vi "Labspec2Matlab.vi"() -> ()   [LabVIEW 2014]
uses:
  Hardware Control/Spectrometer/Spectrometer Function.ctl
  Save Data/SaveData Function.ctl
  Save Data/SaveData Workspace Info.ctl
  <vilib>/regexp/Match Regular Expression.xnode
panel:
  in  "Convert":bool
  in  "Labspec File":path
  # "LICENSED MATERIALS – PROPERTY OF IBM\nCopyright IBM Corp. 2016,\nALL RIGHTS RESERVED"
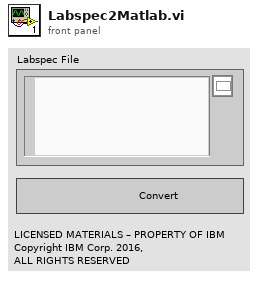
[diagram p1: front panel]
types:
  T1 = typedef "SaveData Function.ctl" = enum16{"Start Python Session", "Set Data Structures to Default", "Append Stress Data", "Append Electrical Measurement", "Append Optical Spectrum", "Append Stress Measurement Step", "Append Instrument Sequence Step", "Set Instrument Configuration", "Set Stress Data", "Set Electrical Measurement", "Set Optical Spectum", "Save Electrical Measurement", "Save Optical Spectrum", "Save Optoelectronic Measurement", "Save Instrument Sequence", "Save Stress Measurement", "Pickle2Workspace", "Explore Variable Space", "Close"}
  T2 = typedef "Spectrometer Function.ctl" = enum16{"Connect", "Complete Configuration", "Get Status", "Load Configuration", "Save Configuration", "Acquire Spectrum", "Read File", "Set Laser", "Set Filter", "Set Hole", "Set Grating", "Set Grating Position", "Set Detector", "Set Acquisition Mode", "Update Refnums", "Disconnect"}
  T3 = typedef "SaveData Workspace Info.ctl" = cluster{"Device Name":string, "Device Info":string, "Path":path}
  T4 = typedef "Spectral Data.ctl" = cluster{"Intensity":dbl[], "Wavelength":dbl[], "Energy":dbl[], "Raman Shift":dbl[], "Detector Temperature":dbl}
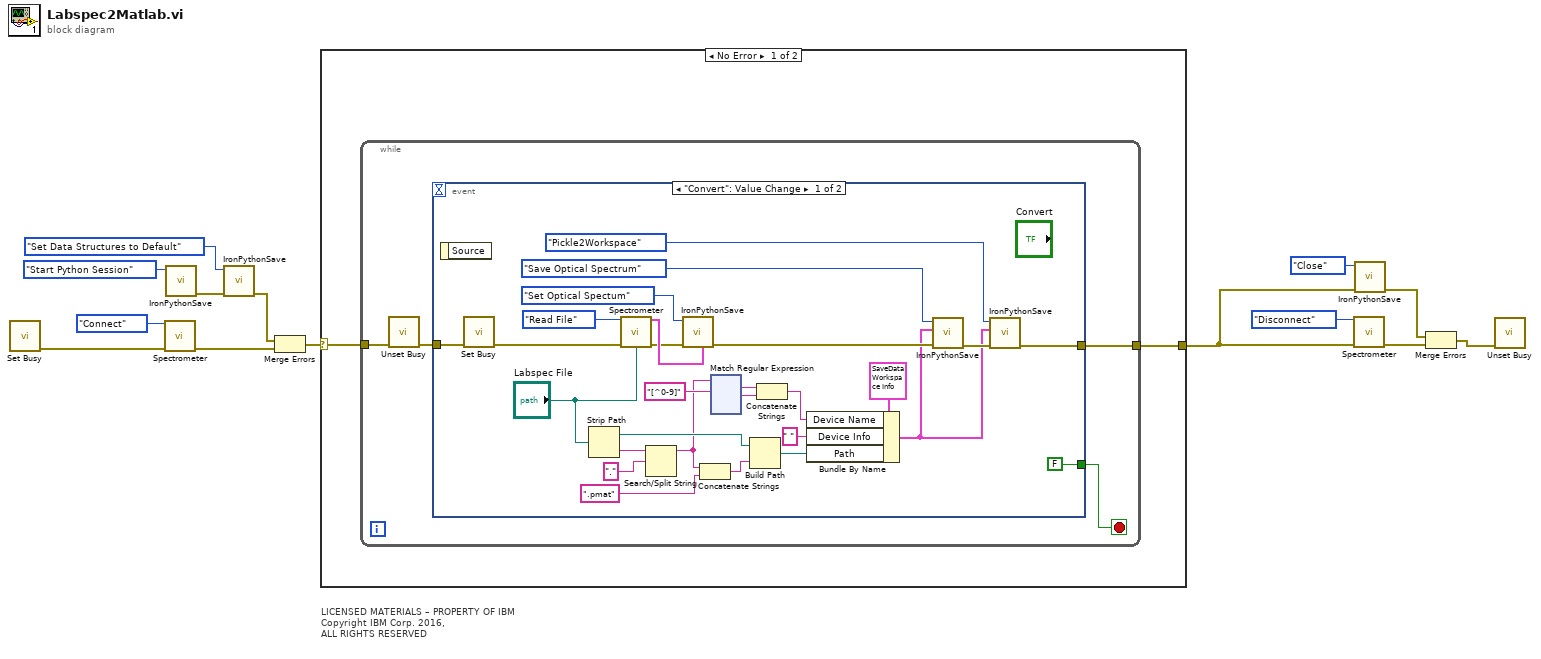
[diagram p0: block diagram]
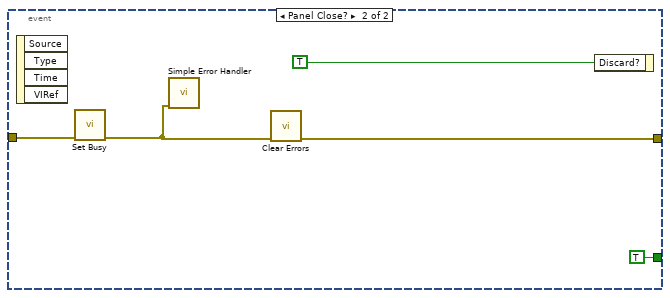
[diagram p2: hidden frame]
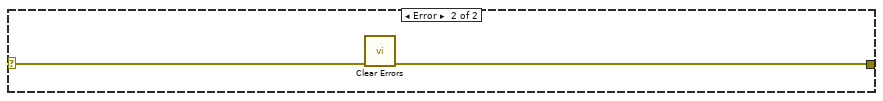
[diagram p3: hidden frame]
diagram:
  # "LICENSED MATERIALS – PROPERTY OF IBM\nCopyright IBM Corp. 2016,\nALL RIGHTS RESERVED"
  n1 = call <vilib>:"Set Busy.vi"() -> ("error out"=w4:errorcluster)  [unwired: 10 in, 1 out]
  n2 = call "Spectrometer.vi"("Function"=Spectrometer_Function."Connect", "error in"=w4) -> ("error out"=w13:errorcluster)  [unwired: 9 in, 4 out]
  n3 = call "IronPythonSave.vi"("Function"=SaveData_Function."Start Python Session") -> ("error out"=w6:errorcluster)  [unwired: 10 in]
  n4 = call "IronPythonSave.vi"("error in (no error)"=w6, "Function"=SaveData_Function."Set Data Structures to Default") -> ("error out"=w5:errorcluster)  [unwired: 9 in]
  n5 = Merge Errors(w5, w13) -> (w11:errorcluster)
  n6 = case shown="No Error" w11 {
    selector: w11 -> [w16 w168]
    tunnel: [w15 w167] -> w8
    frame No Error {
      n7 = while {
        tunnel: w16 -> [w18]
        tunnel: [w20] -> w15
        stop <- w19 stop-if-true
        n8 = call <vilib>:"Unset Busy.vi"("error in (no error)"=w18) -> ("error out"=w17:errorcluster)  [unwired: 10 in]
        n9 = event shown="[0] \"Convert\": Value Change" {
          selector: _ -> [_ _]
          dyn-events: _ -> [_ _]
          timeout: _ -> [_ _]
          tunnel: w17 -> [w27 w165]
          tunnel: [w38 w164] -> w20
          tunnel: [FALSE TRUE] -> w19
          event "Convert": Value Change {
            n10 = event-data() -> ()  [unwired: 1 in, 1 out]
            n11 = call <vilib>:"Set Busy.vi"("error in (no error)"=w27) -> ("error out"=w26:errorcluster)  [unwired: 9 in, 1 out]
            n12 = Strip Path(path="Labspec File") -> (stripped path=w35:path, name=w33:string)
            n13 = call "Spectrometer.vi"("Function"=Spectrometer_Function."Read File", "error in"=w26, "Path"="Labspec File") -> ("Spectrum"=w44:T4, "error out"=w41:errorcluster)  [unwired: 8 in, 3 out]
            n14 = Search/Split String(string=w33, search string/char (-)=".") -> (substring before match=w21:string)  [unwired: 3 out]
            n15 = call "IronPythonSave.vi"("Optical Spectrum"=w44, "error in (no error)"=w41, "Function"=SaveData_Function."Set Optical Spectum") -> ("error out"=w40:errorcluster)  [unwired: 8 in]
            n16 = Concatenate Strings(w21, ".pmat" ("search string/char (-)")) -> (w30:string)
            n17 = xnode "Match Regular Expression"("input string"=w21, "regular expression"="[^0-9]") -> ("whole match"=w24:string, "after match"=w25:string)  [unwired: 4 in, 3 out]
            n18 = Build Path(base path=w35, name or relative path=w30) -> (appended path=w28:path)
            n19 = Concatenate Strings(w24, w25) -> (w23:string)
            n20 = Bundle By Name(cluster=T3 {"Device Name"="test", "Device Info"="test", "Path"=path "C:/Users/gio/Desktop/test Python2Workspace/python2workspace_test.pmat"} ("Workspace Info"), "Device Name"=w23, "Device Info"=" ", "Path"=w28) -> (w32:T3)
            n21 = call "IronPythonSave.vi"("error in (no error)"=w40, "Workspace Info"=w32, "Function"=SaveData_Function."Save Optical Spectrum") -> ("error out"=w39:errorcluster)  [unwired: 8 in]
            n22 = call "IronPythonSave.vi"("error in (no error)"=w39, "Workspace Info"=w32, "Function"=SaveData_Function."Pickle2Workspace") -> ("error out"=w38:errorcluster)  [unwired: 8 in]
          }
          event Panel Close? {
            n23 = event-data() -> ()  [unwired: 1 in, 4 out]
            n24 = call <vilib>:"Set Busy.vi"("error in (no error)"=w165) -> ("error out"=w162:errorcluster)  [unwired: 9 in, 1 out]
            n25 = call <vilib>:"Simple Error Handler.vi"("error in (no error)"=w162) -> ()  [unwired: 4 in, 5 out]
            n26 = call <vilib>:"Clear Errors.vi"("error in (no error)"=w162) -> ("error out"=w164:errorcluster)  [unwired: 5 in, 1 out]
            n27 = event-data("Discard?"=TRUE) -> ()  [unwired: 1 in, 1 out]
          }
        }
      }
    }
    frame Error {
      n28 = call <vilib>:"Clear Errors.vi"("error in (no error)"=w168) -> ("error out"=w167:errorcluster)  [unwired: 5 in, 1 out]
    }
  }
  n29 = call "Spectrometer.vi"("Function"=Spectrometer_Function."Disconnect", "error in"=w8) -> ("error out"=w3:errorcluster)  [unwired: 9 in, 4 out]
  n30 = call "IronPythonSave.vi"("error in (no error)"=w8, "Function"=SaveData_Function."Close") -> ("error out"=w1:errorcluster)  [unwired: 9 in]
  n31 = Merge Errors(w1, w3) -> (w2:errorcluster)
  n32 = call <vilib>:"Unset Busy.vi"("error in (no error)"=w2) -> ()  [unwired: 10 in, 1 out]
